vi "Write ActorMap.vi"(8 "error in (no error)":errorcluster, 10 "ActorMap.lvclass":refnum<class "ActorMap.lvclass">, 11 "Enqueues Data in":refnum<class "Enqueues Data.lvclass">) -> (0 "error out":errorcluster, 3 "Enqueues Data out":refnum<class "Enqueues Data.lvclass">)   [LabVIEW 2020, in "MMVVM Framework.lvlib" / "Enqueues Data.lvclass"]
uses:
  Enqueues Data.lvclass
  ActorMap/ActorMap.lvclass
  Enqueues Data.lvclass/Enqueues Data.ctl
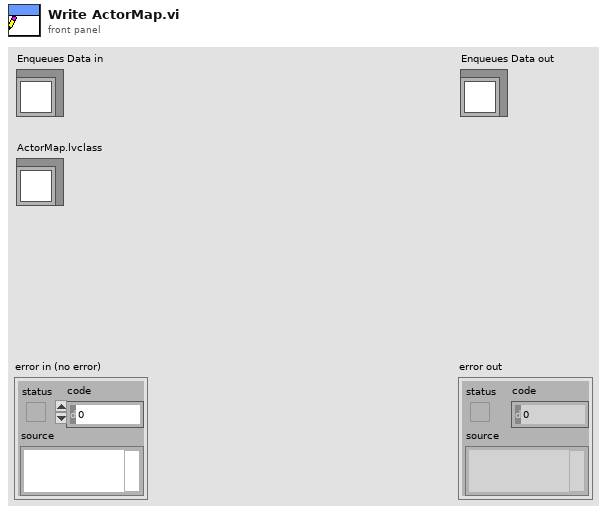
[diagram p1: front panel]
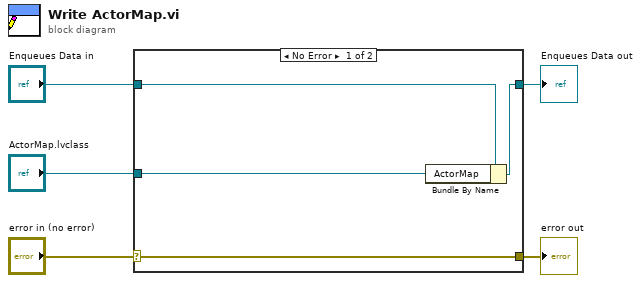
[diagram p0: block diagram]
diagram:
  n1 = case shown="No Error" "error in (no error)" {
    selector: "error in (no error)" -> [w9 w10]
    tunnel: [w9 w10] -> w4
    tunnel: [w7 w11] -> w2
    tunnel: "Enqueues Data in" -> [w8 w11]
    tunnel: "ActorMap.lvclass" -> [w6 _]
    frame No Error {
      n2 = Bundle By Name(cluster=w8, "ActorMap"=w6) -> (w7:refnum<class "Enqueues Data.lvclass">)
    }
    frame Error {
    }
  }
  "error out" <- w4
  "Enqueues Data out" <- w2
